vi "TEST Drop In Cluster.vi"() -> (0 "Cluster":T1)   [LabVIEW 2011]
doc: "This is the cluster for the TEST VI for the drop ins exercise.\n\nAAL 9/09"
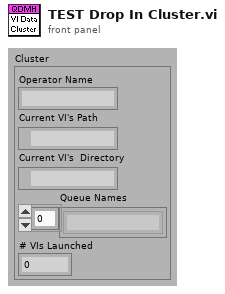
[diagram p1: front panel]
types:
  T1 = cluster{"Operator Name":string, "Current VI's Path":path, "Current VI's  Directory":path, "Queue Names":string[], "# VIs Launched":i32}
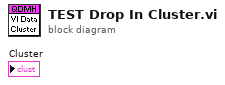
[diagram p0: block diagram]
diagram:
